vi "Open Examples.vi"   [LabVIEW 2023, in "Iterator Actor.lvlib"]
uses:
  Iterator Actor.lvlib
panel:
  # "Run this VI to open the \"Iterator Actor Palette\""
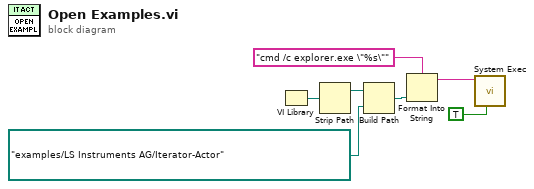
[diagram p0: block diagram]
diagram:
  n1 = VI Library() -> (path=w7:path)
  n2 = Strip Path(path=w7) -> (stripped path=w3:path)  [unwired: 1 out]
  n3 = Build Path(base path=w3, name or relative path=path "examples/LS Instruments AG/Iterator-Actor") -> (appended path=w4:path)
  n4 = Format Into String(format string="cmd /c explorer.exe \"%s\"", w4) -> (resulting string=w2:string)  [unwired: 2 in, 1 out]
  n5 = call <vilib>:"System Exec.vi"("run minimized? (F)"=TRUE, "command line"=w2) -> ()  [unwired: 6 in, 4 out]
